vi "Recurse Cluster or Array.vi"(8 "Skip Outer Cluster":bool, 9 "Cluster or Array":variant, 10 "Lookup String":string, 11 "PropertyObject":refnum<k7>) -> (0 "error out":errorcluster)   [LabVIEW 2020, in "HTS.lvlib" / "VariableContainer.lvclass"]
uses:
  VariableContainer.lvclass
  <vilib>/Utility/Data Type/NI_Data Type.lvlib
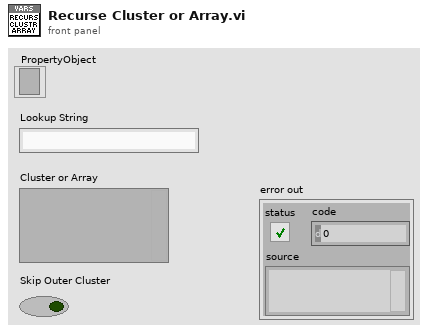
[diagram p1: front panel]
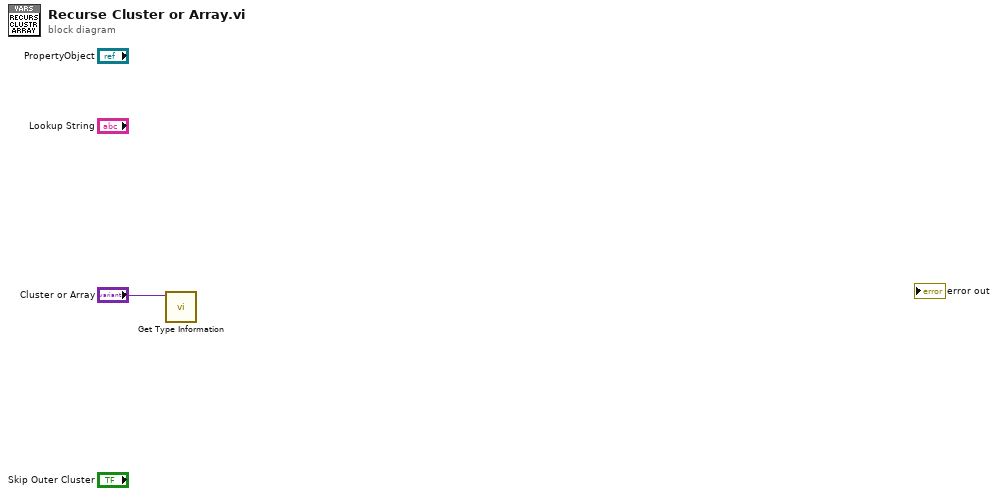
[diagram p0: block diagram]
diagram:
  n1 = call <vilib>:"Get Type Information.vi"("variant"="Cluster or Array") -> ()  [unwired: 6 in, 5 out]
